vi "server.vi"() -> ()   [LabVIEW 2016]
panel:
  out "Dato array":bool[](array[boolean])
  in  "stop":bool
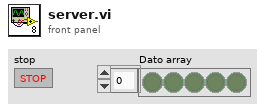
[diagram p1: front panel]
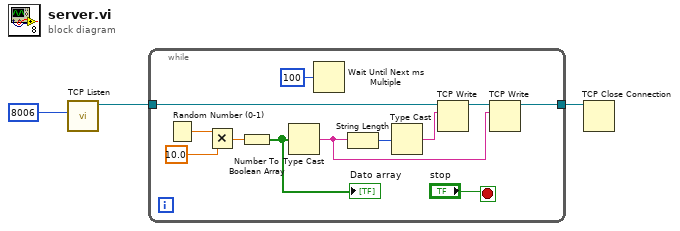
[diagram p0: block diagram]
diagram:
  n1 = call <vilib>:"TCP Listen.vi"("port"=u16 8006) -> ("connection ID"=w3:refnum<k5>)  [unwired: 6 in, 4 out]
  n2 = while {
    tunnel: w3 -> [w15]
    tunnel: [w13] -> w2
    stop <- "stop" stop-if-true
    n3 = Random Number (0-1)() -> (number: 0 to 1=w12:dbl)
    n4 = Multiply(x=w12, y=10.0) -> (x*y=w10:dbl)
    n5 = Number To Boolean Array(number=w10) -> (Boolean array=w9:bool[])
    "Dato array" <- w9
    n6 = Type Cast(x=w9) -> (*(type *) &x=w6:string)  [unwired: 1 in]
    n7 = Wait Until Next ms Multiple(millisecond multiple=u32 100) -> ()  [unwired: 1 out]
    n8 = String Length(string=w6) -> (length=w7:i32)
    n9 = Type Cast(x=w7) -> (*(type *) &x=w8:string)  [unwired: 1 in]
    n10 = TCP Write(connection ID=w15, data in=w8) -> (connection ID out=w14:refnum<k5>)  [unwired: 2 in, 2 out]
    n11 = TCP Write(connection ID=w14, data in=w6) -> (connection ID out=w13:refnum<k5>)  [unwired: 2 in, 2 out]
  }
  n12 = TCP Close Connection(connection ID=w2) -> ()  [unwired: 2 in, 2 out]
